vi "Get Option Value.vi"(8 "error in (no error)":errorcluster, 10 "Option Key":string, 11 "Option Set in":refnum<class "Option Set.lvclass">) -> (0 "error out":errorcluster, 1 "Set":bool, 2 "Value":string, 3 "Option Set out":refnum<class "Option Set.lvclass">)   [LabVIEW 2015, in "Option Parser.lvlib" / "Option Set.lvclass"]
doc: "Get an option based on it's tag.\n<b>Set</b> means the user included it in the parameters.\n<b>Value</b> is the value assigned if it is a value type object."
uses:
  Option Set.lvclass
  Option Set.lvclass/Option Set.ctl
  Option Class/Option.lvclass
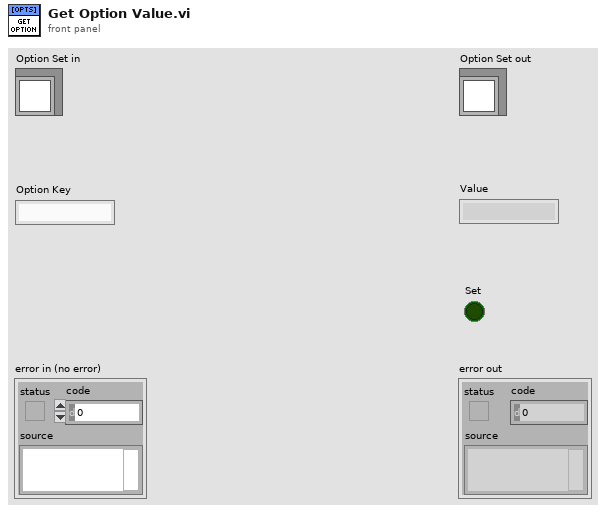
[diagram p1: front panel]
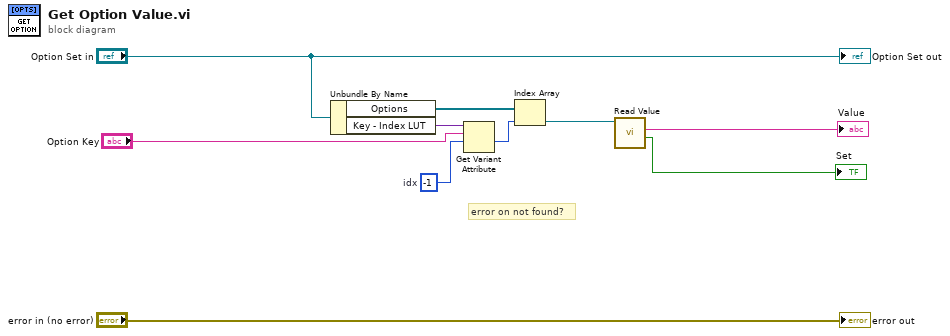
[diagram p0: block diagram]
diagram:
  w4 = -1  # idx
  # "error on not found?"
  n1 = Unbundle By Name("Option Set in") -> ("Options"=w3:refnum<class "Option.lvclass">[], "Key - Index LUT"=w5:variant)
  n2 = Get Variant Attribute(Variant=w5, name="Option Key", default value (empty Variant)=w4) -> (value=w2:i32)  [unwired: 1 in, 3 out]
  n3 = Index Array(array=w3, index=w2) -> (element=w1:refnum<class "Option.lvclass">)
  n4 = call "Read Value.vi"("Option in"=w1) -> ("Set"=→"Set":bool, "Value"=→"Value":string)  [unwired: 8 in, 1 out]
  "error out" <- "error in (no error)"
  "Option Set out" <- "Option Set in"
